vi "saveControls.vi"(7 "prevName":string caption="default name", 8 "error in (no error)":errorcluster, 9 "isAutoSave":bool, 10 "ConfigXMLControls":T1, 11 "ControlsToSave":refnum<vi>[](array[refnum])) -> (0 "error out":errorcluster, 3 "nameUsed":string caption="default name")   [LabVIEW 2015]
uses:
  ConfigXMLControl.ctl
  <vilib>/NI/GXML/GXML.lvlib
panel:
  in  "FILE_NAME":string
  # "Saves the selected controls to an XML file. This will save an XML file\nin the selected directory named ConfigName, or prompt the user for\na name if it is blank. In autosave mode, this saves it into the autosave\ndirectory, in a subdirectory for the current date, and named after the \ncurrent timestamp."
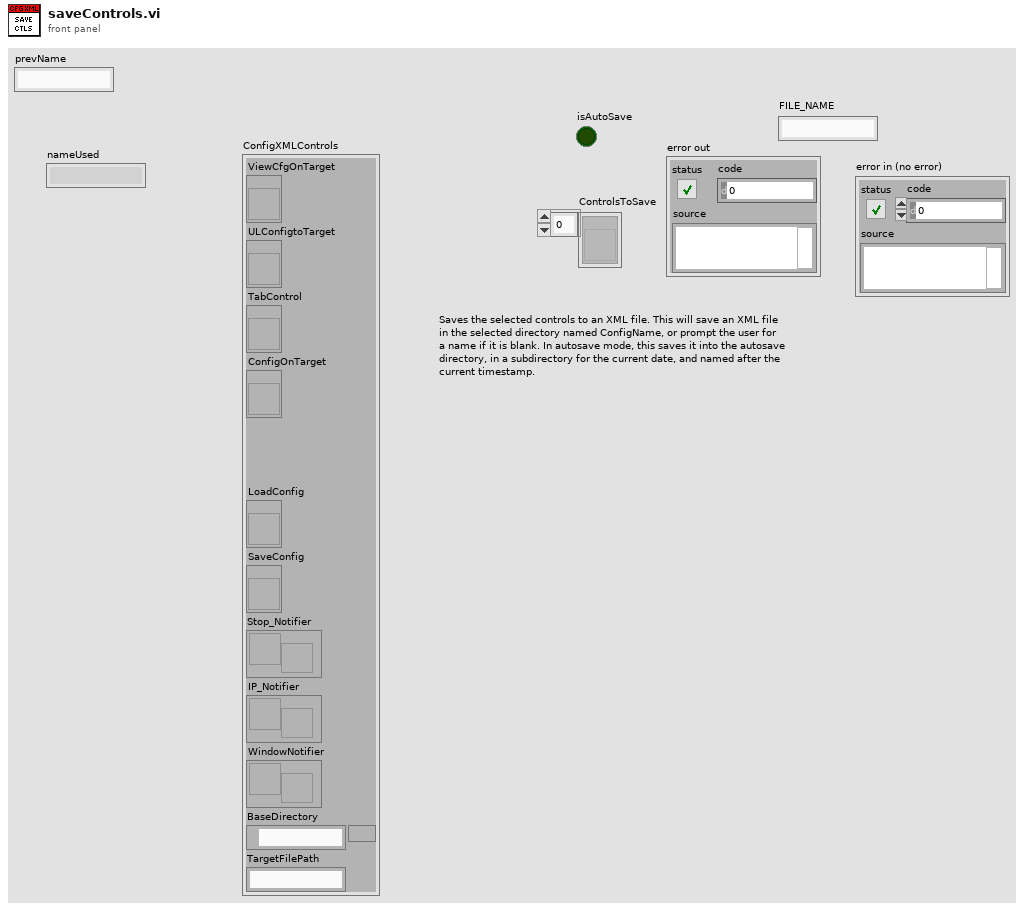
[diagram p1: front panel]
types:
  T1 = typedef "ConfigXMLControl.ctl" = cluster{"ViewCfgOnTarget":refnum<vi>, "ULConfigtoTarget":refnum<vi>, "TabControl":refnum<vi>, "ConfigOnTarget":refnum<vi>, "LoadConfig":refnum<vi>, "SaveConfig":refnum<vi>, "Stop_Notifier":refnum<notifier>, "IP_Notifier":refnum<notifier>, "WindowNotifier":refnum<notifier>, "BaseDirectory":path, "TargetFilePath":string}
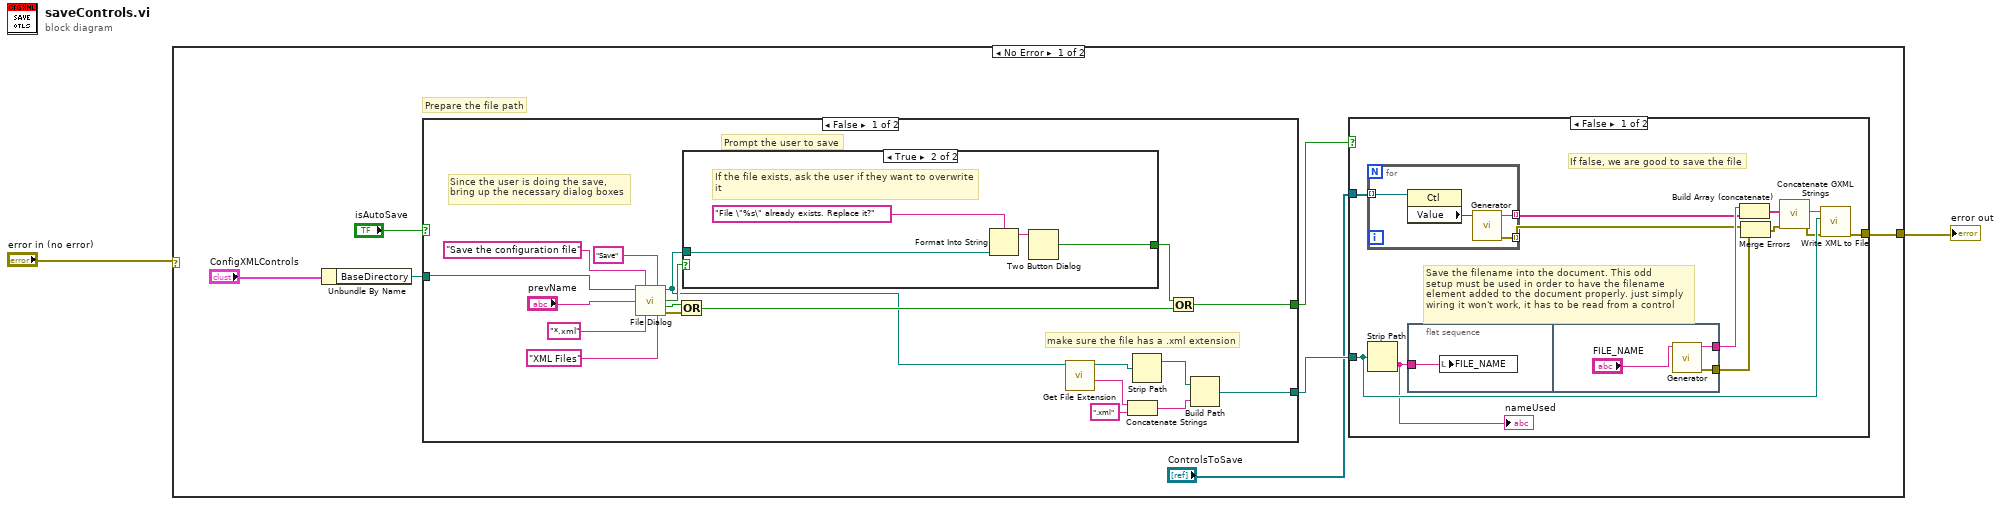
[diagram p0: block diagram]
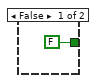
[diagram p3: hidden frame]
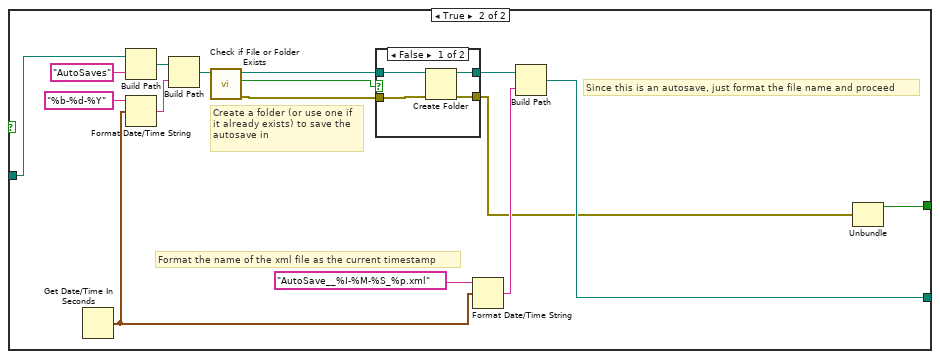
[diagram p4: hidden frame]
diagram:
  n1 = case shown="No Error" "error in (no error)" {
    selector: "error in (no error)" -> [_ w75]
    tunnel: [w3 w75] -> w2
    frame No Error {
      # "Prepare the file path"
      n2 = Unbundle By Name("ConfigXMLControls") -> ("BaseDirectory"=w7:path)
      n3 = case shown="False" "isAutoSave" {
        tunnel: w7 -> [w31 w57]
        tunnel: [w30 w54] -> w6
        tunnel: [w32 w58] -> w5
        frame False {
          # "make sure the file has a .xml extension"
          # "Since the user is doing the save, \nbring up the necessary dialog boxes"
          # "Prompt the user to save"
          n4 = call "File Dialog"("start path"=w31, "prompt"="Save the configuration file", "button label"="Save", "default name"="prevName", "pattern (all files)"="*.xml", "pattern label"="XML Files") -> ("selected path"=w38:path, "exists"=w44:bool, "cancelled"=w43:bool, "error out"=w42:errorcluster)  [unwired: 6 in]
          n5 = Or(x=w43, y=w42) -> (x .or. y?=w40:bool)
          n6 = case shown="True" w44 {
            tunnel: w38 -> [_ w52]
            tunnel: [FALSE ("T button?") w50] -> w41
            frame False {
            }
            frame True {
              # "If the file exists, ask the user if they want to overwrite\nit"
              n7 = Format Into String(format string="File \"%s\" already exists. Replace it?", w52) -> (resulting string=w51:string)  [unwired: 2 in, 1 out]
              n8 = Two Button Dialog(message=w51) -> (T button?=w50:bool)  [unwired: 2 in]
            }
          }
          n9 = call <vilib>:"Get File Extension.vi"("file"=w38) -> ("filename without extension"=w36:string, "dup file"=w37:path)  [unwired: 6 in, 3 out]
          n10 = Concatenate Strings(w36, ".xml" ("string")) -> (w33:string)
          n11 = Strip Path(path=w37) -> (stripped path=w34:path)  [unwired: 1 out]
          n12 = Or(x=w41, y=w40) -> (x .or. y?=w30:bool)
          n13 = Build Path(base path=w34, name or relative path=w33) -> (appended path=w32:path)
        }
        frame True {
          # "Format the name of the xml file as the current timestamp"
          # "Create a folder (or use one if\nit already exists) to save the\nautosave in"
          # "Since this is an autosave, just format the file name and proceed"
          n14 = Get Date/Time In Seconds() -> (seconds since 1Jan1904=w67:timestamp)
          n15 = Build Path(base path=w57, name or relative path="AutoSaves") -> (appended path=w65:path)
          n16 = Format Date/Time String(time format string (%c)="%b-%d-%Y", seconds (now)=w67) -> (date/time string=w64:string)  [unwired: 1 in]
          n17 = Build Path(base path=w65, name or relative path=w64) -> (appended path=w63:path)
          n18 = call <vilib>:"Check if File or Folder Exists.vi"("path"=w63) -> ("error out"=w56:errorcluster, "file or folder exists?"=w62:bool, "dup path"=w61:path)  [unwired: 8 in]
          n19 = case shown="False" w62 {
            tunnel: w61 -> [w73 w74]
            tunnel: [w72 w74] -> w60
            tunnel: [w71 _] -> w55
            tunnel: w56 -> [w70 _]
            frame False {
              n20 = Create Folder(path (use dialog)=w73, error in=w70) -> (created path=w72:path, error out=w71:errorcluster)  [unwired: 1 in, 1 out]
            }
            frame True {
            }
          }
          n21 = Format Date/Time String(time format string (%c)="AutoSave__%I-%M-%S_%p.xml", seconds (now)=w67) -> (date/time string=w59:string)  [unwired: 1 in]
          n22 = Build Path(base path=w60, name or relative path=w59) -> (appended path=w58:path)
          n23 = Unbundle(w55) -> ("status"=w54:bool)  [unwired: 2 out]
        }
      }
      n24 = case shown="False" w6 {
        tunnel: w5 -> [w16 _]
        tunnel: "ControlsToSave" -> [w21 _]
        tunnel: [w12 _] -> w3
        frame False {
          # "If false, we are good to save the file"
          # "Save the filename into the document. This odd\nsetup must be used in order to have the filename\nelement added to the document properly. just simply\nwiring it won't work, it has to be read from a control"
          n25 = for {
            tunnel: w21 -> [w25] mode=indexing
            tunnel: [w23] -> w19 mode=indexing
            tunnel: [w22] -> w15 mode=indexing
            n26 = property class="Ctl"(reference=w25) -> ("Value"=w24:variant)  [unwired: 1 in, 2 out]
            n27 = call <vilib>:"Generator.vi"("Variant"=w24) -> ("error out"=w22:errorcluster, "XML String Out"=w23:string)  [unwired: 9 in]
          }
          n28 = Strip Path(path=w16) -> (name=w10:string)  [unwired: 1 out]
          "nameUsed" <- w10
          n29 = flat-sequence {
            tunnel: w10 -> [w26]
            tunnel: [w28] -> w20
            tunnel: [w27] -> w11
            frame #0 {
              n30 = local write "FILE_NAME"(w26) -> ()
            }
            frame #1 {
              n31 = call <vilib>:"Generator.vi"("Variant"="FILE_NAME") -> ("error out"=w27:errorcluster, "XML String Out"=w28:string)  [unwired: 9 in]
            }
          }
          n32 = Build Array (concatenate)(w20, w19) -> (w18:string[])
          n33 = Merge Errors(w15, w11) -> (w14:errorcluster)
          n34 = call <vilib>:"Concatenate GXML Strings.vi"("error in"=w14, "GXML Strings"=w18) -> ("error out"=w13:errorcluster, "Concatenated GXML String"=w17:string)  [unwired: 8 in]
          n35 = call <vilib>:"Write XML to File.vi"("error in"=w13, "XML File Path"=w16, "XML Input"=w17) -> ("error out"=w12:errorcluster)  [unwired: 8 in]
        }
        frame True {
          # "If true, then the save was either declined by the user, or there was some other error,\nso do not save the file"
        }
      }
    }
    frame Error {
    }
  }
  "error out" <- w2
